vi "Write Listening TS.vi"(8 "error in (no error)":errorcluster, 10 "Listening":u64, 11 "CIFCorePlugin in":refnum<class "CIFCorePlugin.lvclass">) -> (0 "error out":errorcluster, 3 "CIFCorePlugin out":refnum<class "CIFCorePlugin.lvclass">)   [LabVIEW 2021, in "CIFCorePlugin.lvclass"]
doc: "Update the timestamp. Time is U64, absolute time in nS in the appropriate clockID configured for the plugin. If a 0 is wired it will automatically get the current time."
uses:
  CIFCorePlugin.lvclass
  CIFCorePlugin.lvclass/CIFCorePlugin.ctl
  CIFUtilities/CIFClocks/Time Conversion/LabVIEW Time to UTC Time.vi
  CIFUtilities/CIFClocks/SubVIs/Add Error.vi
  CIFUtilities/CIFClocks/CIFClocks.lvlib
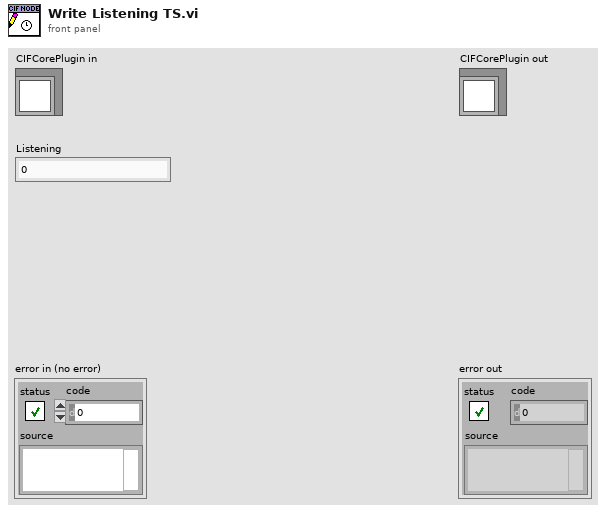
[diagram p1: front panel]
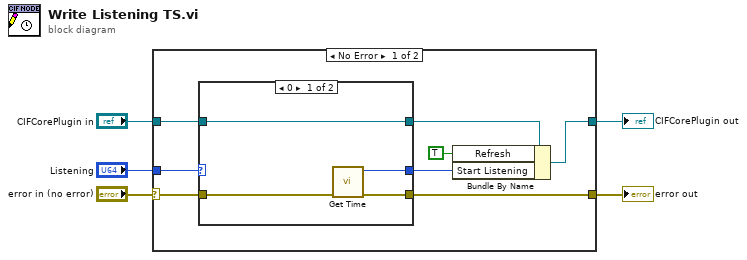
[diagram p0: block diagram]
diagram:
  n1 = case shown="No Error" "error in (no error)" {
    selector: "error in (no error)" -> [w11 w21]
    tunnel: [w7 w21] -> w4
    tunnel: [w13 w22] -> w2
    tunnel: "CIFCorePlugin in" -> [w10 w22]
    tunnel: "Listening" -> [w12 _]
    frame No Error {
      n2 = case shown="0" w12 {
        selector: w12 -> [_ w19]
        tunnel: w11 -> [w17 w18]
        tunnel: w10 -> [w14 w20]
        tunnel: [w14 w20] -> w9
        tunnel: [w16 w19] -> w8
        tunnel: [w15 w18] -> w7
        frame 0 {
          n3 = call "Get Time.vi"("error in (no error)"=w17) -> ("error out"=w15:errorcluster, "Time (ns)"=w16:u64)  [unwired: 8 in, 1 out]
        }
        frame 1, Default {
        }
      }
      n4 = Bundle By Name(cluster=w9, "Refresh"=TRUE, "Start Listening"=w8) -> (w13:refnum<class "CIFCorePlugin.lvclass">)
    }
    frame Error {
    }
  }
  "error out" <- w4
  "CIFCorePlugin out" <- w2
